vi "Rename Templates.vi"(8 "error in (no error)":errorcluster, 9 "Icon Color":u32(colorbox)=13631442, 10 "VI Refs":refnum<vi>[](array[refnum]), 11 "Subsystem Name":string) -> (0 "error out":errorcluster)   [LabVIEW 2019]
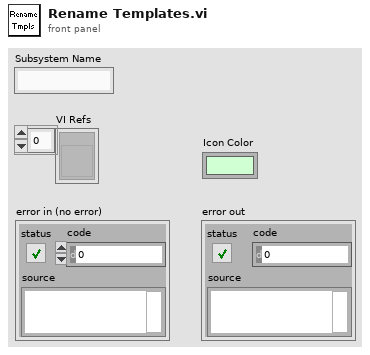
[diagram p1: front panel]
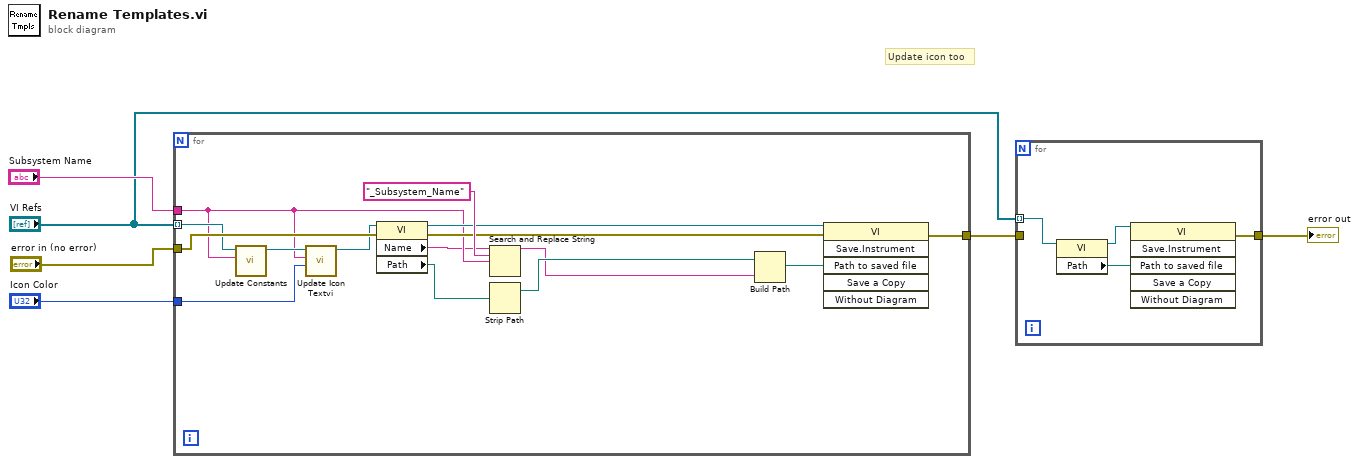
[diagram p0: block diagram]
diagram:
  # "Update icon too"
  n1 = for {
    tunnel: "VI Refs" -> [w13] mode=indexing
    tunnel: "error in (no error)" -> [w16]
    tunnel: "Subsystem Name" -> [w11]
    tunnel: [w15] -> w1
    tunnel: "Icon Color" -> [w10]
    n2 = call <resource>:"Update Constants.vi"("Subsystem Name"=w11, "VI in"=w13) -> ("VI out"=w12:refnum<vi>)  [unwired: 9 in]
    n3 = call <resource>:"Update Icon Textvi.vi"("Icon Color"=w10, "Suubsystem Name"=w11, "vi reference"=w12) -> ("VI Refnum out"=w8:refnum<vi>)  [unwired: 8 in]
    n4 = property class="VI"(reference=w8, error in=w16) -> (reference out=w14:refnum<vi>, error out=w17:errorcluster, "Name"=w9:string, "Path"=w7:path)
    n5 = Search and Replace String(input string=w9, search string="_Subsystem_Name", replace string=w11) -> (result string=w19:string)  [unwired: 5 in, 3 out]
    n6 = Strip Path(path=w7) -> (stripped path=w20:path)  [unwired: 1 out]
    n7 = Build Path(base path=w20, name or relative path=w19) -> (appended path=w18:path)
    n8 = invoke class="VI" method="Save.Instrument"(reference=w14, error in=w17, "Path to saved file"=w18) -> (error out=w15:errorcluster)  [unwired: 3 in, 5 out]
  }
  n9 = for {
    tunnel: [w25] -> w3
    tunnel: "VI Refs" -> [w23] mode=indexing
    tunnel: w1 -> [_]
    n10 = property class="VI"(reference=w23) -> (reference out=w22:refnum<vi>, "Path"=w24:path)  [unwired: 1 in, 1 out]
    n11 = invoke class="VI" method="Save.Instrument"(reference=w22, "Path to saved file"=w24) -> (error out=w25:errorcluster)  [unwired: 4 in, 5 out]
  }
  "error out" <- w3
